vi "31pt Mov Avg.vi"(10 "Value in":dbl) -> (2 "Value out":dbl)   [LabVIEW 2014]
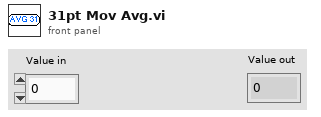
[diagram p1: front panel]
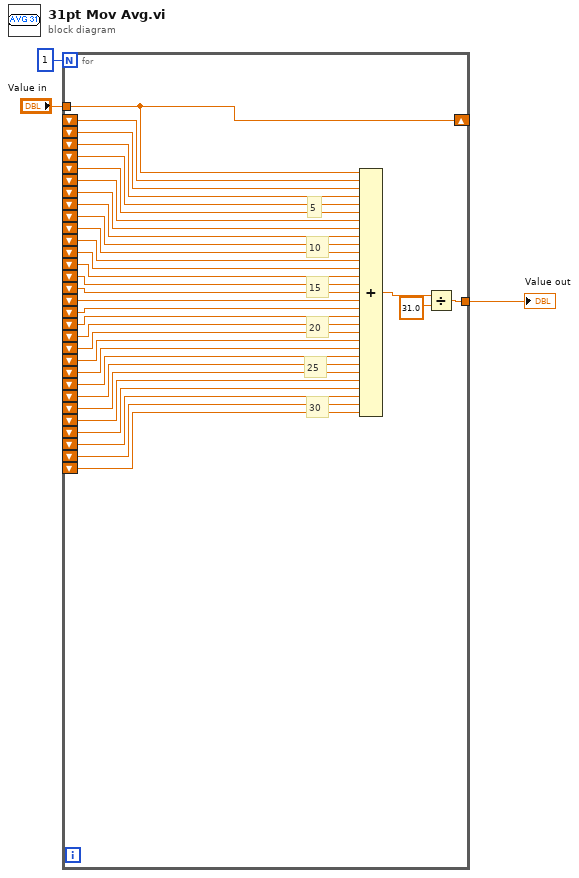
[diagram p0: block diagram]
diagram:
  n1 = for {
    N: 1 -> [_]
    tunnel: "Value in" -> [w37]
    shift-right: [w37] -> _
    shift-left: _ -> [w36]
    shift-left: _ -> [w35]
    shift-left: _ -> [w34]
    shift-left: _ -> [w33]
    tunnel: [w30] -> w1
    shift-left: _ -> [w29]
    shift-left: _ -> [w28]
    shift-left: _ -> [w27]
    shift-left: _ -> [w26]
    shift-left: _ -> [w25]
    shift-left: _ -> [w24]
    shift-left: _ -> [w23]
    shift-left: _ -> [w22]
    shift-left: _ -> [w21]
    shift-left: _ -> [w20]
    shift-left: _ -> [w19]
    shift-left: _ -> [w18]
    shift-left: _ -> [w17]
    shift-left: _ -> [w16]
    shift-left: _ -> [w15]
    shift-left: _ -> [w14]
    shift-left: _ -> [w13]
    shift-left: _ -> [w12]
    shift-left: _ -> [w11]
    shift-left: _ -> [w10]
    shift-left: _ -> [w9]
    shift-left: _ -> [w8]
    shift-left: _ -> [w7]
    shift-left: _ -> [w6]
    shift-left: _ -> [w5]
    shift-left: _ -> [w4]
    # "30"
    # "25"
    # "20"
    # "15"
    # "10"
    # "5"
    n2 = Compound Arithmetic op=ADD(w37, w36, w35, w34, w33, w29, w28, w27, w26, w25, w24, w23, w22, w21, w20, w19, w18, w17, w16, w15, w14, w13, w12, w11, w10, w9, w8, w7, w6, w5, w4) -> (w32:dbl)
    n3 = Divide(x=w32, y=31.0) -> (x/y=w30:dbl)
  }
  "Value out" <- w1
